vi "Parse EndSection-Text.vi"(8 "Error In":errorcluster) -> (0 "Error Out":errorcluster)   [LabVIEW 2018, in "Tests.lvlib" / "Parser.lvlib"]
uses:
  Parser.lvlib
  src/Mustache/Public/Tokens/Public/Text/Text.lvclass
  src/Mustache/Public/Tokens/Public/EndSection/EndSection.lvclass
  src/Mustache/Public/Readers/Public/String/String.lvclass
  D:/Users/cfield/Code/Field R&D Services/Mustache/trunk/src/Mustache/Public/Readers/Public/Abstract/Abstract.lvclass
  <vilib>/Utility/LVClass/Get LV Class Name.vi
  src/Mustache/Public/Tokens/Public/Text/Public/Read Content.vi
  <vilib>/addons/_JKI Toolkits/Caraya/classes/Assert/Assert Equal_Variant.vi
  src/Mustache/Public/Tokens/Public/Keyable/Keyable.lvclass
  <vilib>/addons/_JKI Toolkits/Caraya/classes/Test/Test.lvclass
  src/Mustache/Public/Parser/Parser.lvclass
  <vilib>/addons/_JKI Toolkits/Caraya/classes/Assert/Assert.lvclass
  Tests.lvlib
  src/Mustache/Public/Tokens/Public/Abstract/Abstract.lvclass
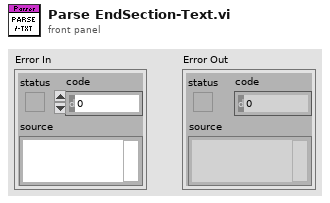
[diagram p1: front panel]
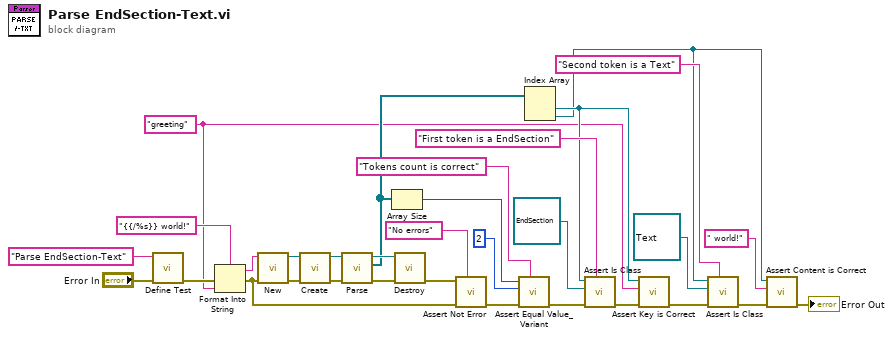
[diagram p0: block diagram]
diagram:
  w4 = "greeting" ("String")
  n1 = call <vilib>:"Define Test.vi"("error in (no error)"="Error In", "Label (VI Title)"="Parse EndSection-Text") -> ("error out"=w23:errorcluster)  [unwired: 9 in]
  n2 = Format Into String(format string="{{/%s}} world!", error in=w23, w4) -> (resulting string=w10:string, error out=w12:errorcluster)  [unwired: 1 in]
  n3 = call "New.vi"("Error In"=w12, "String"=w10) -> ("Error Out"=w29:errorcluster, "String"=w30:refnum<class "String.lvclass">)  [unwired: 8 in]
  n4 = call "Create.vi"("Error In"=w29, "Reader"=w30) -> ("Error Out"=w28:errorcluster, "Parser"=w27:refnum<class "Parser.lvclass">)  [unwired: 8 in]
  n5 = call "Parse.vi"("Error In"=w28, "Parser In"=w27) -> ("Error Out"=w25:errorcluster, "Tokens"=w17:refnum<class "Abstract.lvclass">[], "Parser Out"=w26:refnum<class "Parser.lvclass">)  [unwired: 7 in]
  n6 = Array Size(array=w17) -> (size(s)=w19:i32)
  n7 = call "Destroy.vi"("Error In"=w25, "Parser"=w26) -> ("Error Out"=w24:errorcluster)  [unwired: 9 in]
  n8 = call <vilib>:"Assert Not Error.vi"("Label"="No errors", "error in (no error)"=w12, "Not Error?"=w24) -> ("error out"=w21:errorcluster)  [unwired: 8 in]
  n9 = call <vilib>:"Assert Equal Value_Variant.vi"("Label"="Tokens count is correct", "error in (no error)"=w21, "Y"=2 ("size(s)"), "X"=w19) -> ("error out"=w8:errorcluster)  [unwired: 7 in]
  n10 = Index Array(array=w17) -> (element #1=w5:refnum<class "Abstract.lvclass">, element #2=w2:refnum<class "Abstract.lvclass">)  [unwired: 2 in]
  n11 = call "Assert Is Class.vi"("Label"="First token is a EndSection", "Error In"=w8, "Expected"=refnum<class "EndSection.lvclass"> refnum ("Mustache.lvlib:Tokens.lvlib:EndSection.lvclass"), "Actual"=w5) -> ("Error Out"=w15:errorcluster)  [unwired: 7 in]
  n12 = call "Assert Key is Correct.vi"("Error In"=w15, "Expected"=w4, "Token"=w5) -> ("Error Out"=w7:errorcluster)  [unwired: 8 in]
  n13 = call "Assert Is Class.vi"("Label"="Second token is a Text", "Error In"=w7, "Expected"=refnum<class "Text.lvclass"> refnum ("Mustache.lvlib:Tokens.lvlib:Text.lvclass"), "Actual"=w2) -> ("Error Out"=w13:errorcluster)  [unwired: 7 in]
  n14 = call "Assert Content is Correct.vi"("Error In"=w13, "Expected"=" world!", "Token"=w2) -> ("Error Out"=→"Error Out":errorcluster)  [unwired: 8 in]
